vi "PickedPoint.vi"(8 "error in (no error)":errorcluster, 10 "Point":T2, 11 "Control Window in":refnum<class "Control Window.lvclass">) -> (0 "error out":errorcluster, 1 "Hit?":bool, 2 "PickPoint":T1, 3 "Control Window out":refnum<class "Control Window.lvclass">)   [LabVIEW 2015, in "Control Window.lvclass"]
uses:
  Control Window.lvclass
  <vilib>/Utility/miscctls.llb/LVPoint32TypeDef.ctl
  <vilib>/Utility/miscctls.llb/LV3DPointTypeDef.ctl
  Control Window.lvclass/Control Window.ctl
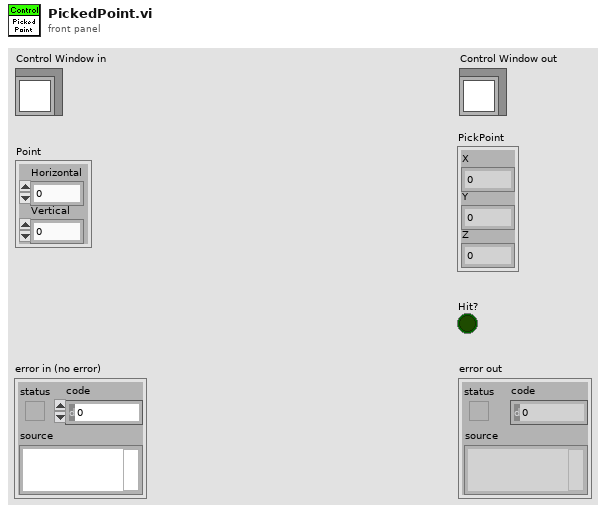
[diagram p1: front panel]
types:
  T1 = typedef "LV3DPointTypeDef.ctl" = cluster{"X":sgl, "Y":sgl, "Z":sgl}
  T2 = typedef "LVPoint32TypeDef.ctl" = cluster{"Horizontal":i32, "Vertical":i32}
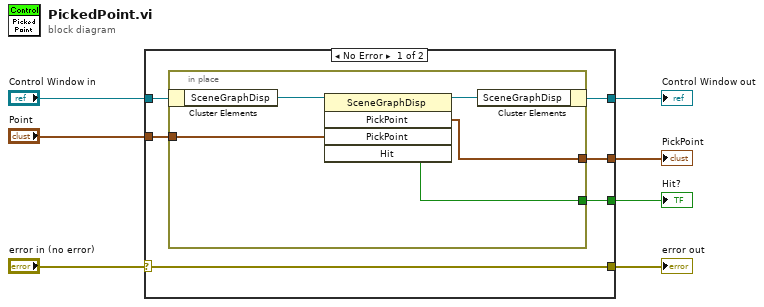
[diagram p0: block diagram]
diagram:
  n1 = case shown="No Error" "error in (no error)" {
    selector: "error in (no error)" -> [w13 w20]
    tunnel: [w13 w20] -> w6
    tunnel: "Control Window in" -> [w12 w19]
    tunnel: [w11 w19] -> w4
    tunnel: "Point" -> [w10 _]
    tunnel: [w9 _] -> w2
    tunnel: [w8 _] -> w1
    frame No Error {
      n2 = in-place {
        in-place-border: w10 -> [w17]
        in-place-border: [w15] -> w9
        in-place-border: [w14] -> w8
        n3 = in-place-cluster #1(w12) -> ("SceneGraphDisp"=w18:refnum<vi>)
        n4 = invoke class="SceneGraphDisp" method="PickPoint"(reference=w18, "PickPoint"=w17) -> (reference out=w16:refnum<vi>, "PickPoint"=w15:T1, "Hit"=w14:bool)  [unwired: 3 in, 2 out]
        n5 = in-place-cluster #1("SceneGraphDisp"=w16) -> (w11:refnum<class "Control Window.lvclass">)
      }
    }
    frame Error {
    }
  }
  "error out" <- w6
  "Control Window out" <- w4
  "PickPoint" <- w2
  "Hit?" <- w1
